vi "振动监测界面.vi"() -> ()   [LabVIEW 2016, in "环境动力监测库.lvlib"]
uses:
  <vilib>/ptbypt/NI_PtbyPt.lvlib
panel:
  out "X4-浸水检测_SJ":bool caption="振动监测"
  # "振动监测"
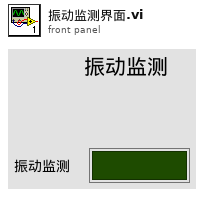
[diagram p1: front panel]
types:
  T1 = cluster{"漏水监测配置":cluster{"监测项描述:输出":string, "端口:":enum16{"AI0", "AI1", "AI2", "AI3", "AI4", "DI0", "DI1", "DI2", "DI3", "DI4", "X0", "X1", "X2", "X3", "X4", "X5", "X6", "X7", "X8", "X9"}, "告警参数:":enum32{"禁用告警", "闭合告警", "断开告警"}, "传感器型号:":enum16{"PLC", "ZLAN"}}, "门禁开关监测配置":cluster{"监测项描述:输出":string, "端口:":enum16{"AI0", "AI1", "AI2", "AI3", "AI4", "DI0", "DI1", "DI2", "DI3", "DI4", "X0", "X1", "X2", "X3", "X4", "X5", "X6", "X7", "X8", "X9"}, "告警参数:":enum32{"禁用告警", "闭合告警", "断开告警"}, "传感器型号:":enum16{"PLC", "ZLAN"}}, "温湿度监测配置":cluster{"监测项描述:输出":string, "端口:":enum16{"AI0", "AI1", "AI2", "AI3", "AI4", "DI0", "DI1", "DI2", "DI3", "DI4", "X0", "X1", "X2", "X3", "X4", "X5", "X6", "X7", "X8", "X9"}, "告警参数:":enum32{"禁用告警", "闭合告警", "断开告警"}, "传感器型号:":enum16{"PLC", "ZLAN"}}, "烟雾监测配置":cluster{"监测项描述:输出":string, "端口:":enum16{"AI0", "AI1", "AI2", "AI3", "AI4", "DI0", "DI1", "DI2", "DI3", "DI4", "X0", "X1", "X2", "X3", "X4", "X5", "X6", "X7", "X8", "X9"}, "告警参数:":enum32{"禁用告警", "闭合告警", "断开告警"}, "传感器型号:":enum16{"PLC", "ZLAN"}}}
  T2 = cluster{"监测项描述:输出":string, "端口:":enum16{"AI0", "AI1", "AI2", "AI3", "AI4", "DI0", "DI1", "DI2", "DI3", "DI4", "X0", "X1", "X2", "X3", "X4", "X5", "X6", "X7", "X8", "X9"}, "告警参数:":enum32{"禁用告警", "闭合告警", "断开告警"}, "传感器型号:":enum16{"PLC", "ZLAN"}}
  T3 = enum16{"AI0", "AI1", "AI2", "AI3", "AI4", "DI0", "DI1", "DI2", "DI3", "DI4", "X0", "X1", "X2", "X3", "X4", "X5", "X6", "X7", "X8", "X9"}
  T4 = cluster{"漏水监测输出":bool, "门禁监测输出":bool, "温湿度监测输出":bool, "烟雾监测输出":bool, "空调监测输出":bool, "自动重合闸输出":bool}
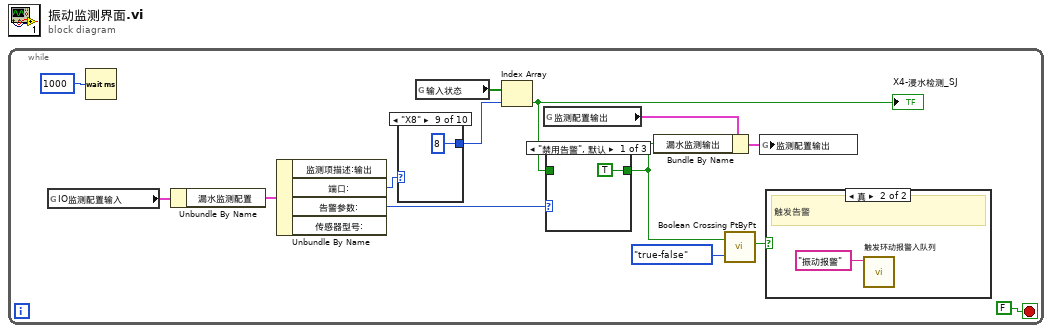
[diagram p0: block diagram]
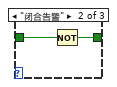
[diagram p3: hidden frame]
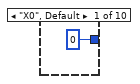
[diagram p5: hidden frame]
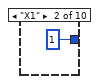
[diagram p6: hidden frame]
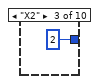
[diagram p7: hidden frame]
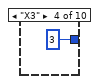
[diagram p8: hidden frame]
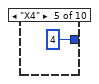
[diagram p9: hidden frame]
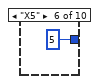
[diagram p10: hidden frame]
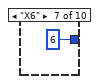
[diagram p11: hidden frame]
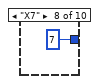
[diagram p12: hidden frame]
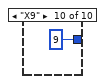
[diagram p13: hidden frame]
diagram:
  n1 = while {
    stop <- FALSE stop-if-true
    n2 = global read "内部交互全局变量.vi" "IO监测配置输入"() -> (w14:T1)
    n3 = Wait (ms)(milliseconds to wait=u32 1000 ("等待时间（毫秒）")) -> ()  [unwired: 1 out]
    n4 = Unbundle By Name(w14) -> ("漏水监测配置"=w13:T2)
    n5 = Unbundle By Name(w13) -> ("端口:"=w12:T3, "告警参数:"=w7:enum32{"禁用告警", "闭合告警", "断开告警"})  [unwired: 2 out]
    n6 = case shown="\"X8\"" w12 {
      tunnel: [0 ("索引") 1 ("索引") 2 ("索引") 3 ("索引") 4 ("索引") 5 ("索引") 6 ("索引") 7 ("索引") 8 ("索引") 9 ("索引")] -> w10
      frame "X0", Default {
      }
      frame "X1" {
      }
      frame "X2" {
      }
      frame "X3" {
      }
      frame "X4" {
      }
      frame "X5" {
      }
      frame "X6" {
      }
      frame "X7" {
      }
      frame "X8" {
      }
      frame "X9" {
      }
    }
    n7 = global read "外部交互全局变量.vi" "输入状态"() -> (w11:bool[])
    n8 = Index Array(array=w11, index=w10) -> (element=w6:bool)
    "X4-浸水检测_SJ" <- w6
    n9 = global read "内部交互全局变量.vi" "监测配置输出"() -> (w9:T4)
    n10 = case shown="\"禁用告警\", 默认" w7 {
      tunnel: w6 -> [_ w18 w19]
      tunnel: [TRUE ("漏水监测输出") w17 w19] -> w1
      frame "禁用告警", Default {
      }
      frame "闭合告警" {
        n11 = Not(x=w18) -> (.not. x?=w17:bool)
      }
      frame "断开告警" {
      }
    }
    n12 = Bundle By Name(cluster=w9, "漏水监测输出"=w1) -> (w8:T4)
    n13 = call <vilib>:"Boolean Crossing PtByPt.vi"("direction"=enum16{"either", "false-true", "true-false"}."true-false", "input"=w1) -> ("crossing"=w2:bool)  [unwired: 1 in]
    n14 = global write "内部交互全局变量.vi" "监测配置输出"(w8) -> ()
    n15 = case shown="真" w2 {
      frame False {
      }
      frame True {
        # "触发告警"
        n16 = call "触发环动报警入队列.vi"("报警内容"="振动报警") -> ()  [unwired: 11 in]
      }
    }
  }
